vi "Update HWI.vi"(3 "Error In":errorcluster, 4 "Current Variables":T1[](array[typedef]), 6 "Devices queue":refnum<queue>) -> (0 "Error Out":errorcluster, 2 "Devices queue out":refnum<queue>)   [LabVIEW 2013]
uses:
  TypeDefs/Active procedure variables.ctl
  Device/Device.lvclass
  Master Device/Master Device.lvclass
panel:
  out "Check HWI Timing":u32[](array[numeric])
  out "Finalize HWI Timing":u32[](array[numeric])
  out "Prep HWI Timing":u32[](array[numeric])
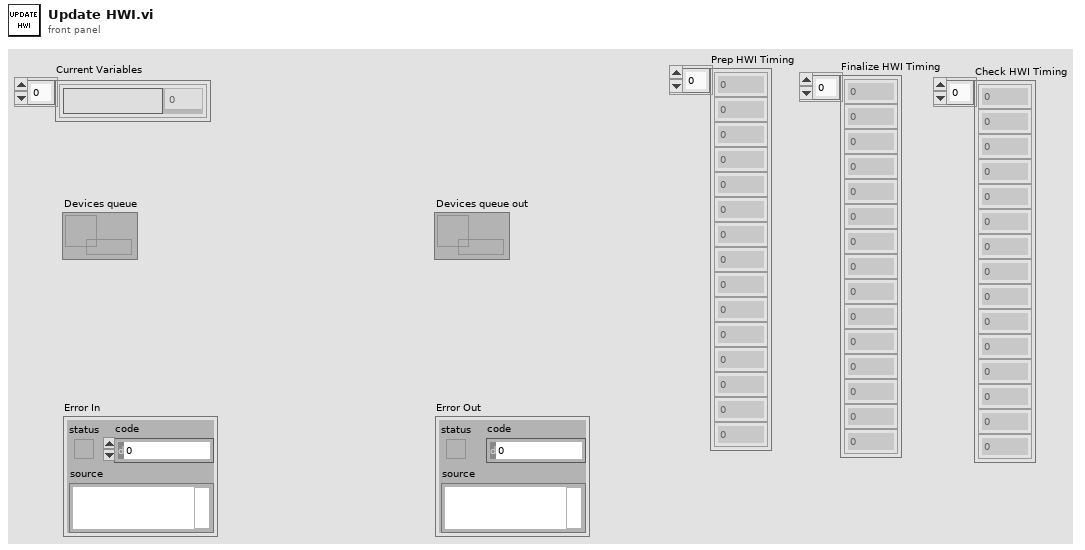
[diagram p1: front panel]
types:
  T1 = typedef "Active procedure variables.ctl" = cluster{"Procedure variable":string, "Value":dbl}
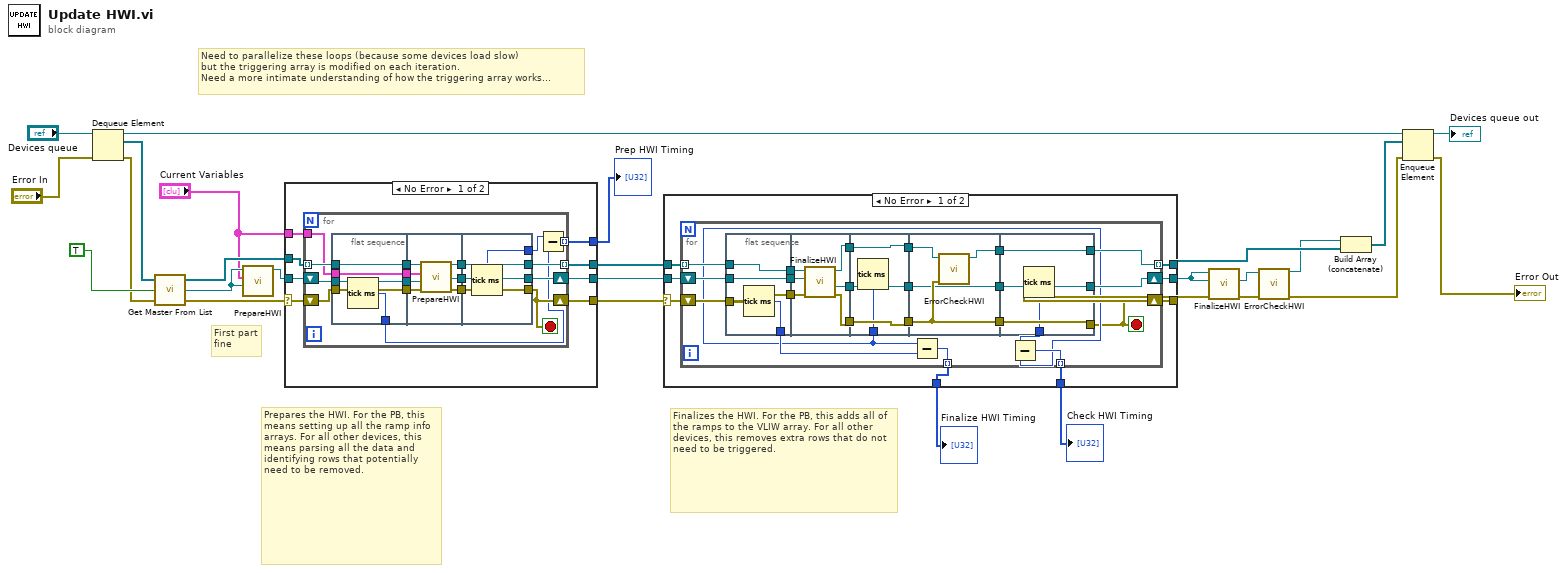
[diagram p0: block diagram]
diagram:
  # "First part\nfine"
  # "Finalizes the HWI. For the PB, this adds all of the ramps to the VLIW array. For all other devices, this removes extra rows that do not need to be triggered."
  # "Prepares the HWI. For the PB, this means setting up all the ramp info arrays. For all other devices, this means parsing all the data and identifying rows that potentially need to be removed."
  # "Need to parallelize these loops (because some devices load slow)\nbut the triggering array is modified on each iteration.\nNeed a more intimate understanding of how the triggering array works..."
  n1 = Dequeue Element(queue="Devices queue", error in (no error)="Error In") -> (queue out=w4:refnum<queue>, element=w8:refnum<class "Device.lvclass">[], error out=w7:errorcluster)  [unwired: 1 in, 1 out]
  n2 = call "Get Master From List.vi"("error in"=w7, "Del From List?"=TRUE, "Device List in"=w8) -> ("error out"=w23:errorcluster, "Master Device"=w21:refnum<class "Master Device.lvclass">, "Device List out"=w24:refnum<class "Device.lvclass">[])
  n3 = call-dynamic "PrepareHWI.vi"(9:"Master Device in"=w21, "Current Variables"="Current Variables", 11:"Master Device in"=w21) -> ("Master Device out"=w20:refnum<class "Master Device.lvclass">)  [unwired: 6 in, 2 out]
  n4 = case shown="No Error" w23 {
    selector: w23 -> [w35 w71]
    tunnel: [w30 w71] -> w27
    tunnel: [w31 w70] -> w26
    tunnel: w24 -> [w32 w70]
    tunnel: w20 -> [w34 w69]
    tunnel: "Current Variables" -> [w33 _]
    tunnel: [w29 w69] -> w18
    tunnel: [w28 _] -> w12
    frame No Error {
      n5 = for {
        shift-right: [w48] -> w30
        shift-left: w35 -> [w49]
        shift-right: [w47] -> w29
        shift-left: w34 -> [w50]
        tunnel: w33 -> [w51]
        tunnel: w32 -> [w52] mode=indexing
        tunnel: [w46] -> w31 mode=indexing
        tunnel: [w36] -> w28 mode=indexing
        stop <- w48 stop-if-true
        n6 = flat-sequence {
          tunnel: w49 -> [w54]
          tunnel: w50 -> [w55]
          tunnel: w51 -> [w56]
          tunnel: w52 -> [w57]
          tunnel: [w57] -> w45
          tunnel: [w56] -> w44
          tunnel: [w55] -> w43
          tunnel: [w54] -> w42
          tunnel: [w53] -> w37
          tunnel: w45 -> [w64]
          tunnel: w44 -> [w63]
          tunnel: w43 -> [w62]
          tunnel: w42 -> [w61]
          tunnel: [w60] -> w41
          tunnel: [w59] -> w40
          tunnel: [w58] -> w39
          tunnel: [w66] -> w46
          tunnel: [w67] -> w47
          tunnel: [w68] -> w48
          tunnel: w41 -> [w68]
          tunnel: w40 -> [w67]
          tunnel: w39 -> [w66]
          tunnel: [w65] -> w38
          frame #0 {
            n7 = Tick Count (ms)() -> (millisecond timer value=w53:u32)
          }
          frame #1 {
            n8 = call-dynamic "PrepareHWI.vi"("error in (no error)"=w61, "Master Device in"=w62, "Current Variables"=w63, "Device in"=w64) -> ("error out"=w60:errorcluster, "Master Device out"=w59:refnum<class "Master Device.lvclass">, "Device out"=w58:refnum<class "Device.lvclass">)  [unwired: 5 in]
          }
          frame #2 {
            n9 = Tick Count (ms)() -> (millisecond timer value=w65:u32)
          }
        }
        n10 = Subtract(x=w38, y=w37) -> (x-y=w36:u32)
      }
    }
    frame Error {
    }
  }
  "Prep HWI Timing" <- w12
  n11 = case shown="No Error" w27 {
    selector: w27 -> [w78 w127]
    tunnel: [w79 w127] -> w17
    tunnel: w26 -> [w77 w126]
    tunnel: [w74 w126] -> w25
    tunnel: w18 -> [w76 w125]
    tunnel: [w75 w125] -> w16
    tunnel: [w73 _] -> w11
    tunnel: [w72 _] -> w10
    frame No Error {
      n12 = for {
        shift-right: [w80] -> w79
        shift-left: w78 -> [w100]
        shift-right: [w92] -> w75
        shift-left: w76 -> [w101]
        tunnel: w77 -> [w102] mode=indexing
        tunnel: [w93] -> w74 mode=indexing
        tunnel: [w84] -> w73 mode=indexing
        tunnel: [w83] -> w72 mode=indexing
        stop <- w80 stop-if-true
        n13 = flat-sequence {
          tunnel: w100 -> [w104]
          tunnel: w101 -> [w105]
          tunnel: w102 -> [w106]
          tunnel: [w106] -> w88
          tunnel: [w105] -> w87
          tunnel: [w104] -> w86
          tunnel: [w103] -> w85
          tunnel: [w109] -> w99
          tunnel: [w108] -> w98
          tunnel: [w107] -> w97
          tunnel: w88 -> [w112]
          tunnel: w87 -> [w111]
          tunnel: w86 -> [w110]
          tunnel: w99 -> [w116]
          tunnel: w98 -> [w115]
          tunnel: w97 -> [w114]
          tunnel: [w116] -> w96
          tunnel: [w115] -> w95
          tunnel: [w114] -> w94
          tunnel: [w113] -> w81
          tunnel: w96 -> [w117]
          tunnel: w95 -> [w119]
          tunnel: w94 -> [w120]
          tunnel: [w120] -> w91
          tunnel: [w118] -> w90
          tunnel: [w117] -> w89
          tunnel: [w122] -> w92
          tunnel: [w123] -> w93
          tunnel: [w124] -> w80
          tunnel: w91 -> [w124]
          tunnel: w90 -> [w123]
          tunnel: w89 -> [w122]
          tunnel: [w121] -> w82
          frame #0 {
            n14 = Tick Count (ms)() -> (millisecond timer value=w103:u32)
          }
          frame #1 {
            n15 = call-dynamic "FinalizeHWI.vi"("error in (no error)"=w110, "Master Device in"=w111, "Device in"=w112) -> ("error out"=w107:errorcluster, "Master Device out"=w109:refnum<class "Master Device.lvclass">, "Device out"=w108:refnum<class "Device.lvclass">)  [unwired: 6 in]
          }
          frame #2 {
            n16 = Tick Count (ms)() -> (millisecond timer value=w113:u32)
          }
          frame #3 {
            n17 = call-dynamic "ErrorCheckHWI.vi"("error in (no error)"=w120, "Device in"=w119) -> ("Device out"=w118:refnum<class "Device.lvclass">)  [unwired: 8 in, 1 out]
          }
          frame #4 {
            n18 = Tick Count (ms)() -> (millisecond timer value=w121:u32)
          }
        }
        n19 = Subtract(x=w81, y=w85) -> (x-y=w84:u32)
        n20 = Subtract(x=w82, y=w81) -> (x-y=w83:u32)
      }
    }
    frame Error {
    }
  }
  "Finalize HWI Timing" <- w11
  "Check HWI Timing" <- w10
  n21 = call-dynamic "FinalizeHWI.vi"("error in (no error)"=w17, 10:"Master Device in"=w16, 11:"Master Device in"=w16) -> ("error out"=w14:errorcluster, "Master Device out"=w15:refnum<class "Master Device.lvclass">)  [unwired: 6 in, 1 out]
  n22 = call-dynamic "ErrorCheckHWI.vi"("error in (no error)"=w14, "Device in"=w15) -> ("error out"=w1:errorcluster, "Device out"=w13:refnum<class "Master Device.lvclass">)  [unwired: 8 in]
  n23 = Build Array (concatenate)(w13, w25) -> (w3:refnum<class "Device.lvclass">[])
  n24 = Enqueue Element(queue=w4, element=w3, error in (no error)=w1) -> (queue out=→"Devices queue out":refnum<queue>, error out=→"Error Out":errorcluster)  [unwired: 1 in, 1 out]
